vi "DB_Query.vi"(8 "error in (no error)":errorcluster, 10 "Parameters":string[](array[string]), 11 "Parameterized Query":string) -> (0 "error out":errorcluster, 2 "Query in Standard Format":string, 3 "Results":variant[][](array[variant]))   [LabVIEW 2013]
uses:
  <vilib>/addons/database/Auxilliary.llb/DB Tools Parameter Info.ctl
  <vilib>/addons/database/Auxilliary.llb/DB Tools DataTypes.ctl
  <vilib>/addons/database/Auxilliary.llb/DB Tools Parameter Dir.ctl
  <userlib>/_OpenG.lib/string/string.llb/Trim Whitespace (String Array)__ogtk.vi
  <vilib>/addons/database/Command.llb/Cmd Execute.vi
  <vilib>/addons/database/Recordset.llb/Rec Fetch Recordset Data (CR).vi
  <vilib>/addons/database/Recordset.llb/Rec Destroy - Command.vi
  <vilib>/addons/database/Command.llb/Cmd Delete.vi
  <vilib>/addons/database/NI_Database_API.lvlib
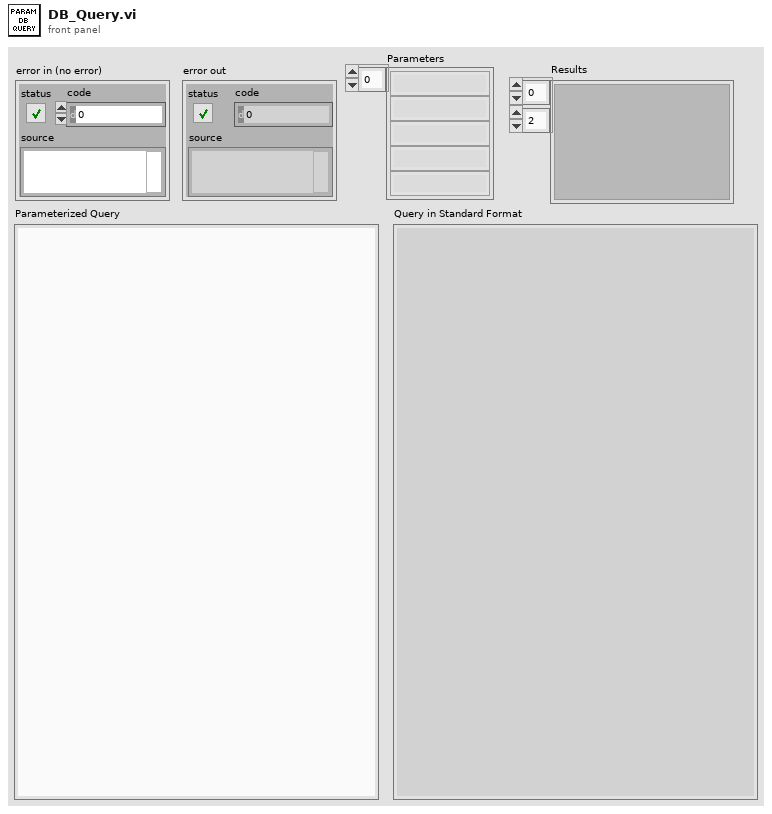
[diagram p1: front panel]
types:
  T1 = typedef "NI_Database_API.lvlib/DB Tools DataTypes.ctl" = enum16{"String", "Long (I32)", "Single (SGL)", "Double (DBL)", "Date/Time", "Binary"}
  T2 = typedef "NI_Database_API.lvlib/DB Tools Parameter Dir.ctl" = enum32{"Input", "Output", "Input/Output", "Return Value"}
  T3 = typedef "NI_Database_API.lvlib/DB Tools Parameter Info.ctl" = cluster{"parameter name":string, "type":T1, "direction":T2, "value":variant}
  T4 = typedef "NI_Database_API.lvlib/Conn ObjectReference.ctl" = refnum<k1>
  T5 = typedef "NI_Database_API.lvlib/Cmd ObjectReference.ctl" = refnum<k1>
  T6 = typedef "NI_Database_API.lvlib/Cmd-Rec Object Reference.ctl" = refnum<k1>
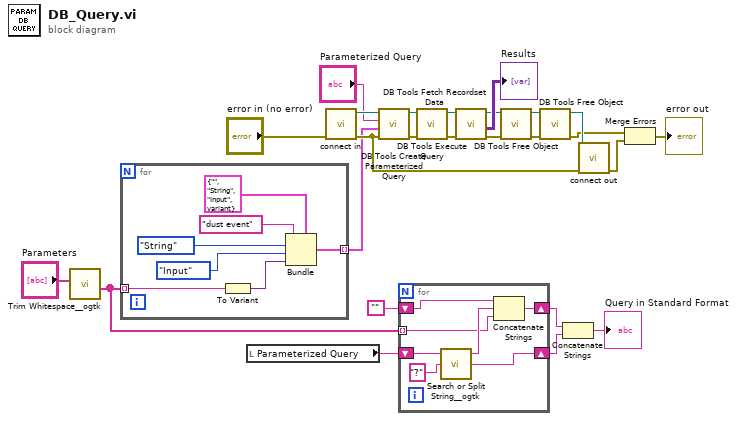
[diagram p0: block diagram]
diagram:
  n1 = call-poly <userlib>:"Trim Whitespace__ogtk.vi"("String in"="Parameters") -> ("String out"=w5:string[])  [unwired: 6 in]
  n2 = for {
    tunnel: [w27] -> w8 mode=indexing
    tunnel: w5 -> [w26] mode=indexing
    n3 = To Variant(anything=w26) -> (Variant=w31:variant)
    n4 = Bundle(cluster=T3 {"parameter name"="", "type"=enum."String", "direction"=enum."Input", "value"=variant} ("parameter information"), "parameter name"="dust event", "type"=DB_Tools_DataTypes."String", "direction"=DB_Tools_Parameter_Dir."Input", "value"=w31) -> (w27:T3)
  }
  n5 = local read "Parameterized Query"() -> (w6:string)
  n6 = call "connect in.vi"("error in (no error)"="error in (no error)") -> ("error out"=w16:errorcluster, "Database Connection"=w15:T4)  [unwired: 6 in, 1 out]
  n7 = call <vilib>:"DB Tools Create Parameterized Query.vi"("error in (no error)"=w16, "parameters"=w8, "SQL query"="Parameterized Query", "connection reference"=w15) -> ("error out"=w17:errorcluster, "command reference"=w14:T5)  [unwired: 3 in, 1 out]
  n8 = for {
    shift-right: [w36] -> w2
    shift-left: w6 -> [w39]
    tunnel: w5 -> [w33] mode=indexing
    shift-right: [w37] -> w3
    shift-left: "" -> [w35]
    n9 = call <userlib>:"Search or Split String__ogtk.vi"("search string/char (-)"="?", "string"=w39) -> ("substring after match"=w36:string, "substring before match"=w34:string)  [unwired: 1 in, 1 out]
    n10 = Concatenate Strings(w35, w34, w33) -> (w37:string)
  }
  n11 = call-poly <vilib>:"DB Tools Execute Query.vi"("error in (no error)"=w17, "command reference"=w14) -> ("error out"=w18:errorcluster, "command-recordset reference"=w19:T6)  [unwired: 6 in]
  n12 = call-poly <vilib>:"DB Tools Fetch Recordset Data.vi"("error in (no error)"=w18, "command-recordset reference"=w19) -> ("error out"=w20:errorcluster, "recordset data"=→"Results":variant[][], "command-recordset reference out"=w21:T6)  [unwired: 3 in]
  n13 = call-poly <vilib>:"DB Tools Free Object.vi"("error in (no error)"=w20, "command-recordset reference"=w21) -> ("error out"=w10:errorcluster, "command reference"=w12:T5)  [unwired: 8 in]
  n14 = call-poly <vilib>:"DB Tools Free Object.vi"("error in (no error)"=w10, "command reference"=w12) -> ("error out"=w9:errorcluster, "connection reference"=w11:T4)  [unwired: 8 in]
  n15 = Concatenate Strings(w3, w2) -> (→"Query in Standard Format":string)
  n16 = call "connect out.vi"("error in (no error)"=w16, "connection reference"=w11) -> ("error out"=w22:errorcluster)  [unwired: 9 in]
  n17 = Merge Errors(w9, w22) -> (→"error out":errorcluster)
